vi "Complete Testing.vi"(8 "error in (no error)":errorcluster, 11 "Context in":refnum<class "Context.lvclass">) -> (0 "error out":errorcluster, 3 "Context out":refnum<class "Context.lvclass">)   [LabVIEW 2015, in "Context.lvclass"]
uses:
  Context.lvclass
  Context.lvclass/Context.ctl
  States/State/State.lvclass
  Model/Model/Model.lvclass
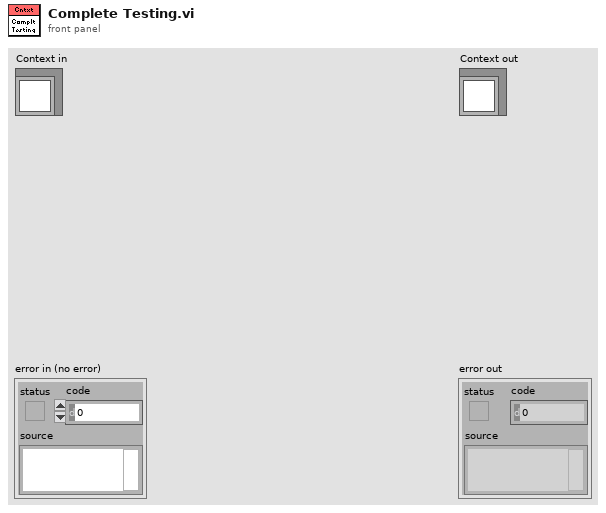
[diagram p1: front panel]
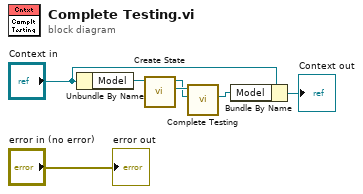
[diagram p0: block diagram]
diagram:
  n1 = Unbundle By Name("Context in") -> ("Model"=w6:refnum<class "Model.lvclass">)
  n2 = call "Create State.vi"("Model in"=w6) -> ("State"=w3:refnum<class "State.lvclass">, "Model out"=w2:refnum<class "Model.lvclass">)  [unwired: 8 in, 1 out]
  n3 = call-dynamic "Complete Testing.vi"("Model in"=w2, "State in"=w3) -> ("Model out"=w1:refnum<class "Model.lvclass">)  [unwired: 7 in, 2 out]
  n4 = Bundle By Name(cluster="Context in", "Model"=w1) -> (→"Context out":refnum<class "Context.lvclass">)
  "error out" <- "error in (no error)"
